vi "Read Module Specific Configuration.vi"(8 "error in":errorcluster, 11 "Standard Engine Configuration in":refnum<class "Standard Engine Configuration.lvclass">) -> (0 "error out":errorcluster, 2 "Module Specific Configuration":T1[](array[typedef]), 3 "Standard Engine Configuration out":refnum<class "Standard Engine Configuration.lvclass">)   [LabVIEW 2013, in "Standard Engine Configuration.lvclass"]
doc: "Returns an array of module specific execution information including module ID, decimation, and error configuration."
uses:
  Standard Engine Configuration.lvclass
  Module Specific Configuration.ctl
  Module Decimation.ctl
  Module Error Configuration.ctl
  Error Actions By Category.ctl
  <vilib>/NI/Tag Bus Module Framework/runtime/error classification.ctl
  Error Actions.ctl
  Standard Engine Configuration.lvclass/Standard Engine Configuration.ctl
  <vilib>/NI/Tag Bus Module Framework/runtime/TBM module execution interface.lvclass
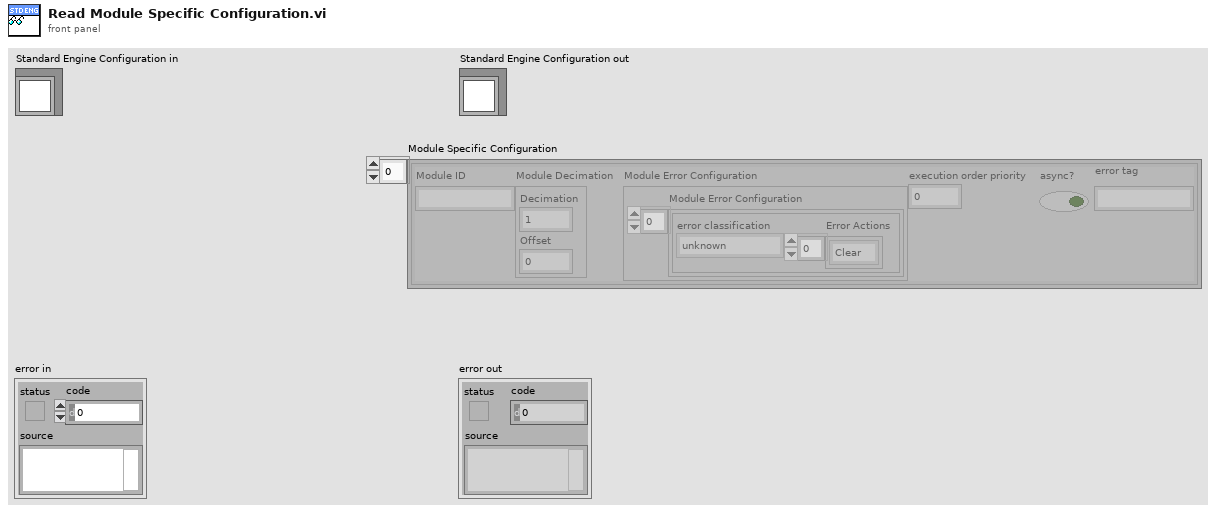
[diagram p1: front panel]
types:
  T1 = typedef "Standard Engine Configuration.lvclass/Module Specific Configuration.ctl" = cluster{"Module ID":string, "Module Decimation":T2, "Module Error Configuration":T3, "execution order priority":i32, "async?":bool, "error tag":string}
  T2 = typedef "Standard Engine Configuration.lvclass/Module Decimation.ctl" = cluster{"Decimation":u16, "Offset":u16}
  T3 = typedef "Standard Engine Configuration.lvclass/Module Error Configuration.ctl" = cluster{"Module Error Configuration":T4[]}
  T4 = typedef "Standard Engine Configuration.lvclass/Error Actions By Category.ctl" = cluster{"error classification":T5, "Error Actions":T6[]}
  T5 = typedef "TBM module execution interface.lvclass/error classification.ctl" = enum16{"unknown", "none", "trivial", "recoverable", "critical"}
  T6 = typedef "Standard Engine Configuration.lvclass/Error Actions.ctl" = enum16{"Clear", "Notify", "Stop Component", "Stop Engine", "Safe State", "Attempt Recovery"}
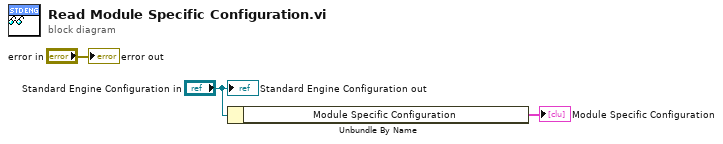
[diagram p0: block diagram]
diagram:
  n1 = Unbundle By Name("Standard Engine Configuration in") -> ("Module Specific Configuration"=→"Module Specific Configuration":T1[])
  "error out" <- "error in"
  "Standard Engine Configuration out" <- "Standard Engine Configuration in"
